vi "FTW-ActorTemplate.vi"(0 "FTW Actor Instance Configuration":string="{\n  \"Identity\": \"ActorName\",\n  \"InboxAddress\": \"inproc://*\",\n  \"LoggerAddress\": \"\",\n  \"DebugEnableInboxLogging\": false,\n  \"DebugEnableJobLogging\": false,\n  \"LauncherAddress\": \"\"\n}", 11 "ErrorIn":errorcluster) -> (15 "Error":errorcluster)   [LabVIEW 2015]
uses:
  source/actor/Instance/FTW-ActorInstance.lvclass
  source/actor/Message/Base/FTW-Message.lvclass
  source/actor/Instance/FTW-ActorInstance.lvclass/FTW-ActorInstance.ctl
  source/actor/JobSequencer/FTW-SEQ-Current.vi
  source/actor/Message/Request/FTW-Message-IncomingRequest.lvclass
panel:
  # "Inputs"
  # "Outputs"
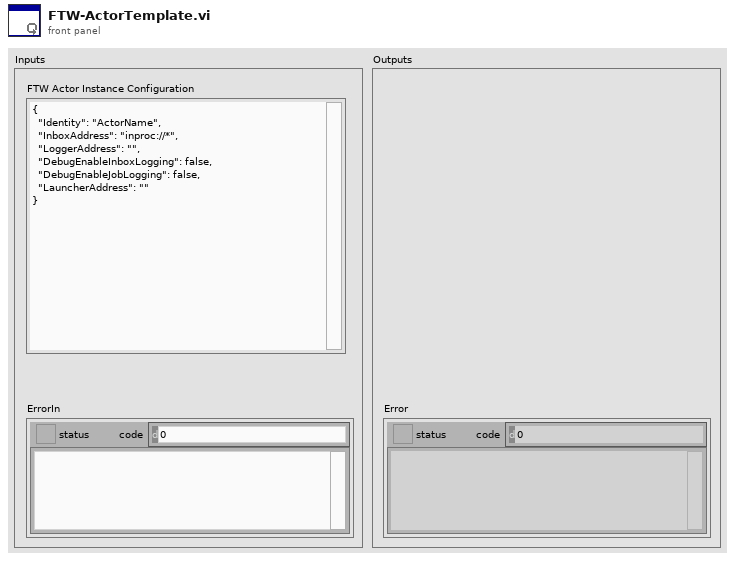
[diagram p1: front panel]
types:
  T1 = cluster{"Incoming Requests":refnum<event-registration>, "Local Messages":refnum<event-registration>, "Additional Registration Types":refnum<event-registration>}
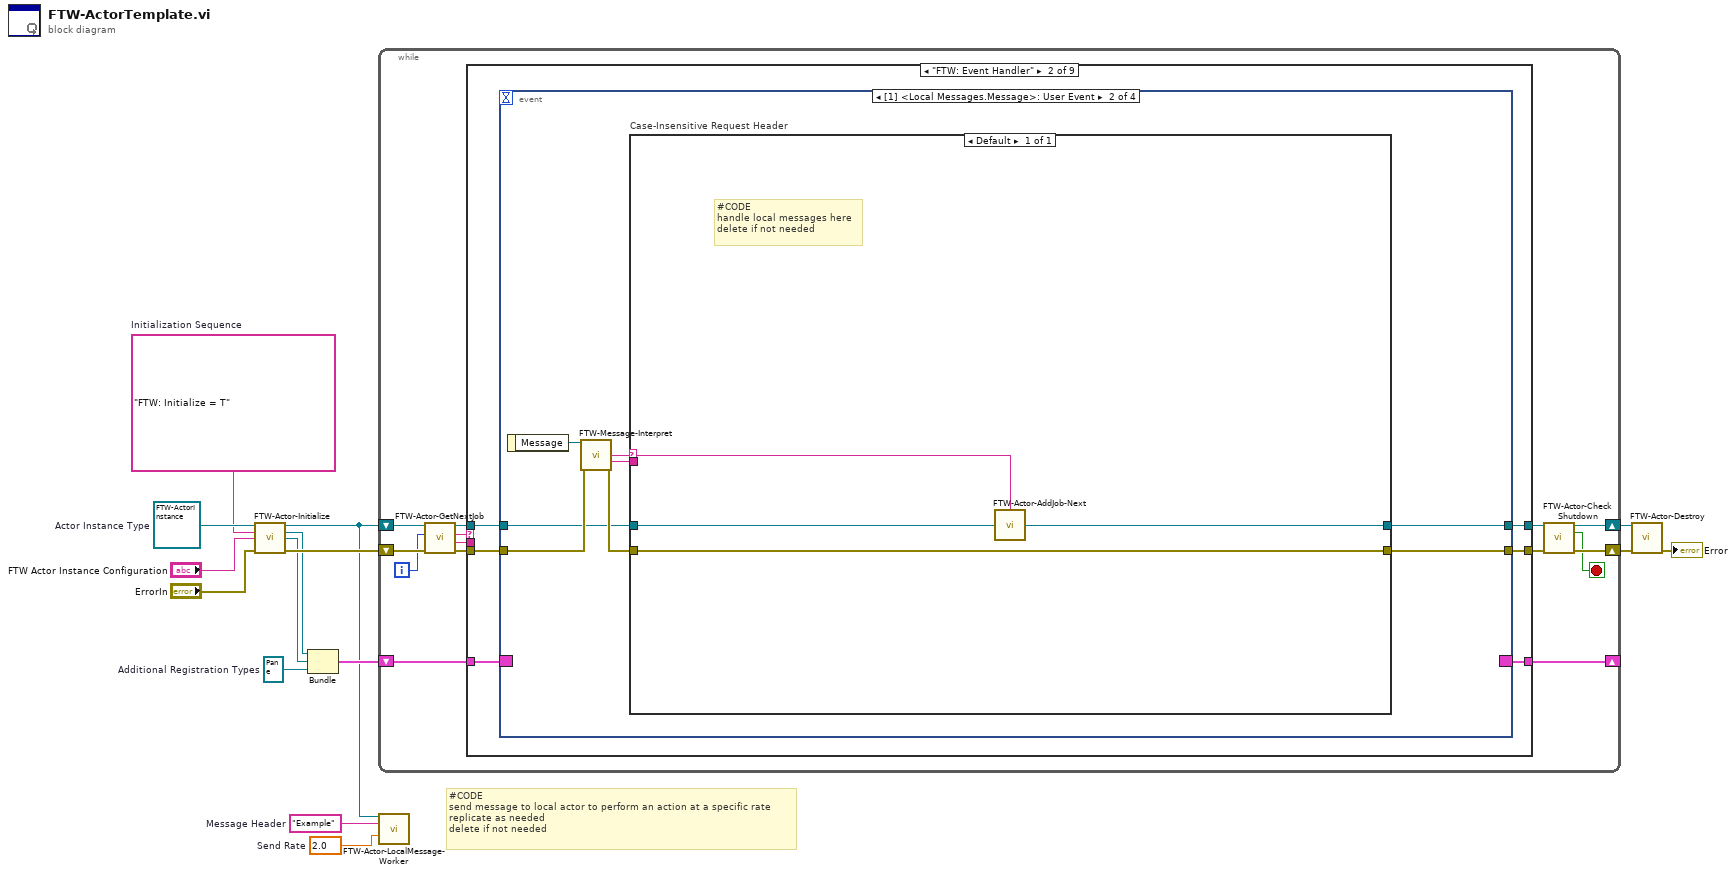
[diagram p0: block diagram]
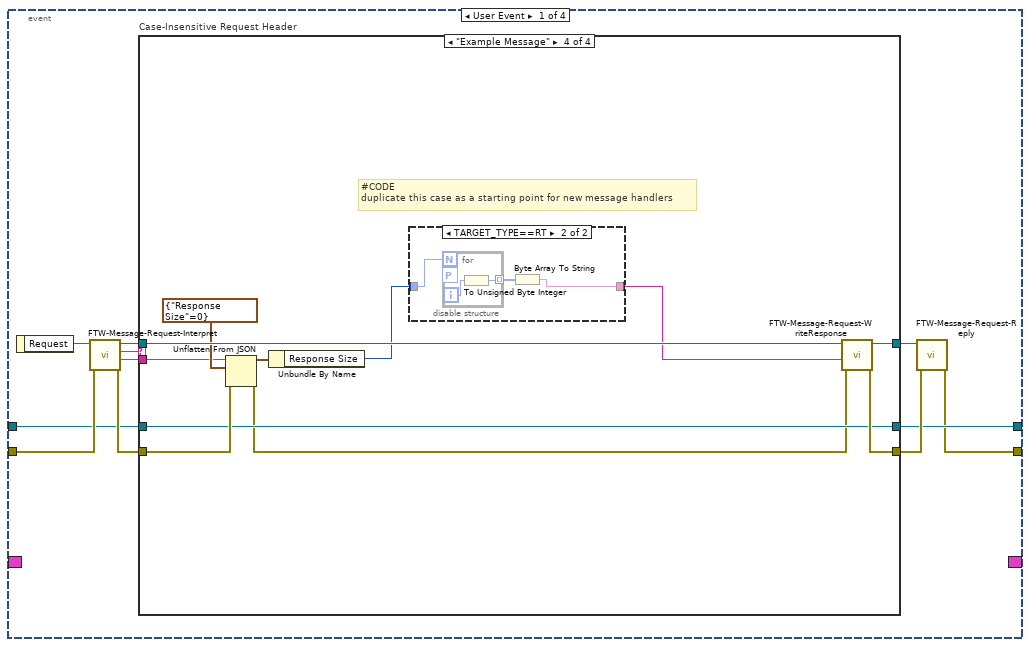
[diagram p3: hidden frame]
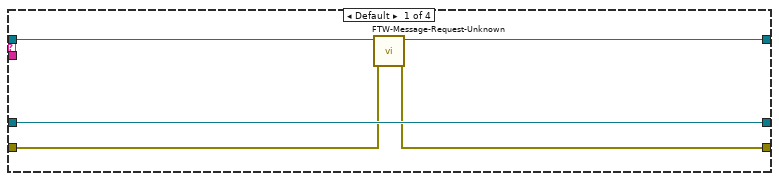
[diagram p4: hidden frame]
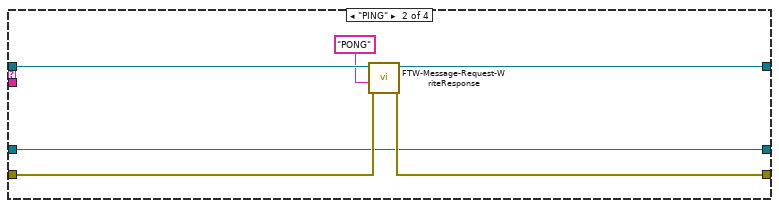
[diagram p5: hidden frame]
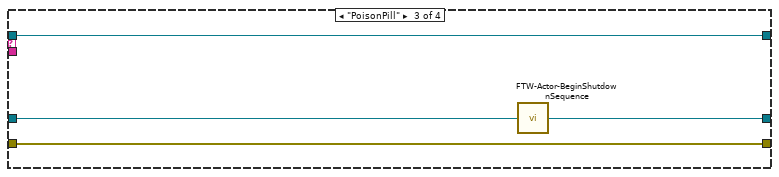
[diagram p6: hidden frame]
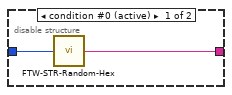
[diagram p7: hidden frame]
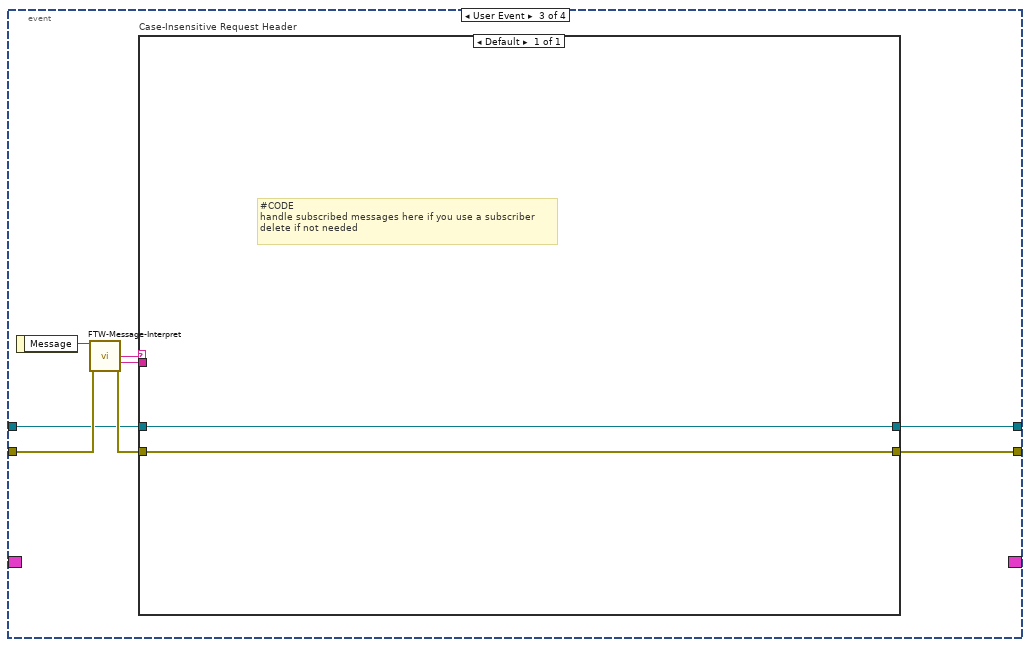
[diagram p8: hidden frame]
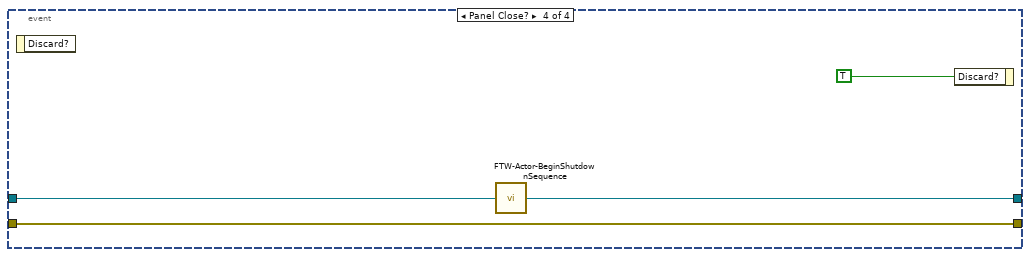
[diagram p9: hidden frame]
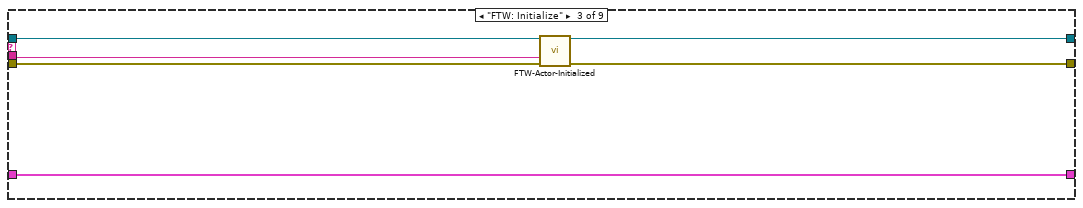
[diagram p10: hidden frame]
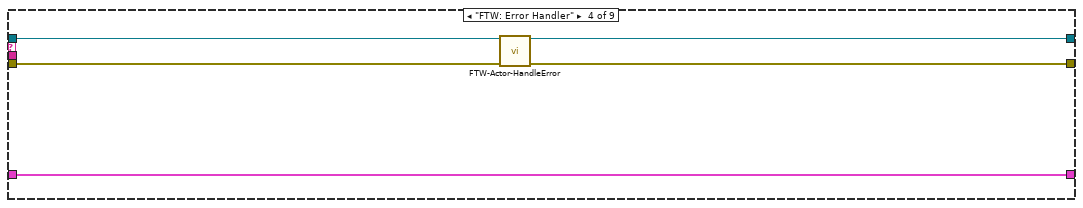
[diagram p11: hidden frame]
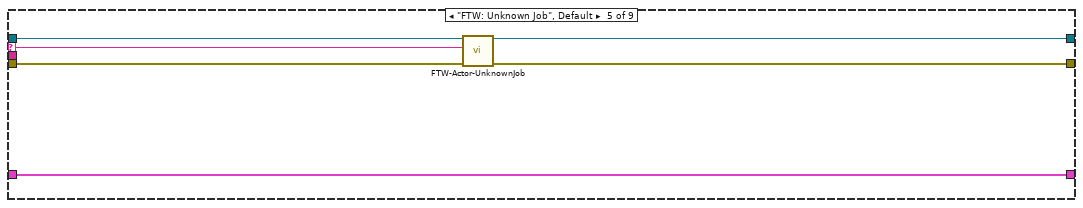
[diagram p12: hidden frame]
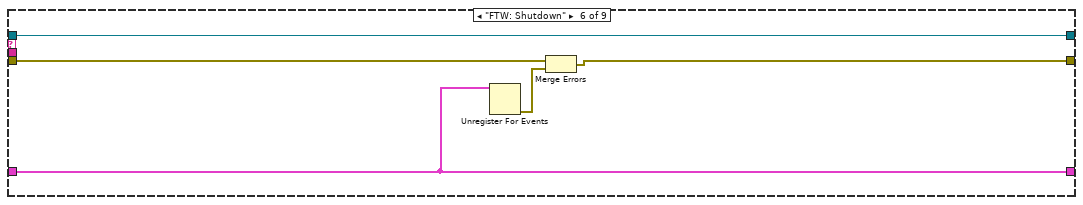
[diagram p13: hidden frame]
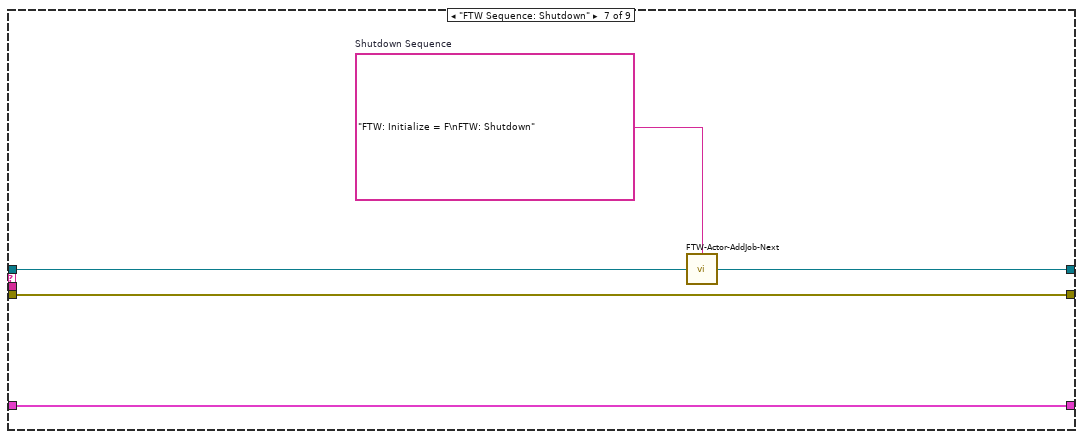
[diagram p14: hidden frame]
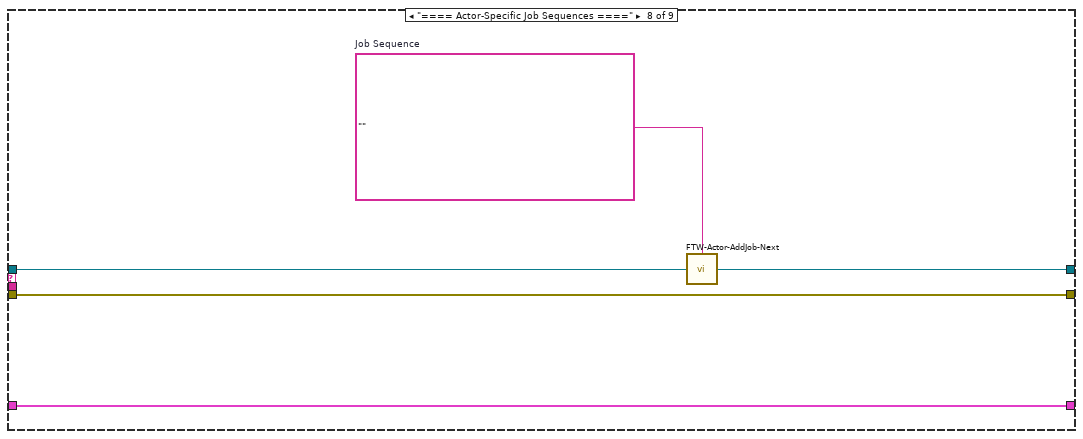
[diagram p15: hidden frame]
diagram:
  w1 = 2.0  # Send Rate
  w2 = "Example"  # Message Header
  w4 = refnum<event-registration> refnum  # Additional Registration Types
  w11 = refnum<class "FTW-ActorInstance.lvclass"> refnum  # Actor Instance Type
  w10 = "FTW: Initialize = T"  # Initialization Sequence
  # "#CODE\nsend message to local actor to perform an action at a specific rate\nreplicate as needed\ndelete if not needed"
  n1 = call-dynamic "FTW-Actor-Initialize.vi"("FTW Actor Instance Type"=w11, "Initialization Job Sequence"=w10, "Actor Instance Configuration"="FTW Actor Instance Configuration", "error in"="ErrorIn") -> ("FTW Actor Instance"=w3:refnum<class "FTW-ActorInstance.lvclass">, "Incoming Requests"=w6:refnum<event-registration>, "Local Messages"=w5:refnum<event-registration>, "error out"=w12:errorcluster)  [unwired: 8 in]
  n2 = Bundle("Incoming Requests"=w6, "Local Messages"=w5, "Additional Registration Types"=w4) -> (w8:T1)  [unwired: 1 in]
  n3 = while {
    shift-right: [w19] -> w14
    shift-left: w12 -> [w26]
    shift-right: [w16] -> _
    shift-left: w8 -> [w29]
    shift-right: [w21] -> w15
    shift-left: w3 -> [w28]
    i -> [w17]
    stop <- w18 stop-if-true
    n4 = call "FTW-Actor-GetNextJob.vi"("error in"=w26, "Jobs Performed"=w17, "FTW Actor Instance"=w28) -> ("error out"=w25:errorcluster, "Job Data"=w23:string, "Job Name"=w24:string, "FTW Actor Instance out"=w27:refnum<class "FTW-ActorInstance.lvclass">)  [unwired: 5 in]
    n5 = case shown="\"FTW: Event Handler\"" w24 {
      selector: w24 -> [_ _ _ _ w120 _ _ _ _]
      tunnel: [w31 w38 w110 w115 w123 w129 w134 w139 w143] -> w20
      tunnel: w25 -> [w31 w37 w113 w117 w124 w130 w134 w139 w143]
      tunnel: w29 -> [w32 w33 w114 w119 w125 w126 w135 w140 w142]
      tunnel: [w32 w36 w114 w119 w125 w126 w135 w140 w142] -> w16
      tunnel: w23 -> [_ _ w109 _ _ _ _ _ _]
      tunnel: [w30 w35 w111 w116 w121 w127 w132 w137 w141] -> w22
      tunnel: w27 -> [w30 w34 w112 w118 w122 w127 w133 w138 w141]
      frame "==== Featherweight Framework Jobs ====" {
      }
      frame "FTW: Event Handler" {
        n6 = event shown="[1] <Local Messages.Message>: User Event" {
          selector: w33 -> [_ _ _ _]
          dyn-events: [_ _ _ _] -> w36
          timeout: _ -> [_ _ _ _]
          tunnel: [w41 w87 w99 w107] -> w38
          tunnel: w37 -> [w47 w88 w100 w107]
          tunnel: [w45 w86 w98 w105] -> w35
          tunnel: w34 -> [w44 w85 w97 w106]
          event User Event {
            n7 = event-data() -> ("Request"=w48:refnum<class "FTW-Message-IncomingRequest.lvclass">)  [unwired: 1 in]
            n8 = call "FTW-Message-Request-Interpret.vi"("error in"=w47, "FTW Incoming Request"=w48) -> ("error out"=w49:errorcluster, "Request Body"=w39:string, "Request Header"=w43:string, "FTW Incoming Request out"=w42:refnum<class "FTW-Message-IncomingRequest.lvclass">)  [unwired: 6 in]
            n9 = case "Case-Insensitive Request Header" shown="\"Example Message\"" w43 {
              tunnel: [w52 w58 w63 w74] -> w46
              tunnel: w49 -> [w53 w59 w63 w75]
              tunnel: [w54 w57 w64 w71] -> w45
              tunnel: w44 -> [w54 w57 w62 w71]
              tunnel: w42 -> [w51 w60 w61 w73]
              tunnel: [w50 w56 w61 w72] -> w40
              tunnel: w39 -> [_ _ _ w65]
              frame Default {
                n10 = call "FTW-Message-Request-Unknown.vi"("error in"=w53, "FTW Incoming Request"=w51) -> ("error out"=w52:errorcluster, "FTW Incoming Request Out"=w50:refnum<class "FTW-Message-IncomingRequest.lvclass">)  [unwired: 8 in]
              }
              frame "PING" {
                n11 = call "FTW-Message-Request-WriteResponse.vi"("error in"=w59, "Response Body"="PONG" ("Response Header"), "FTW Incoming Request"=w60) -> ("error out"=w58:errorcluster, "FTW Incoming Request out"=w56:refnum<class "FTW-Message-IncomingRequest.lvclass">)  [unwired: 7 in]
              }
              frame "PoisonPill" {
                n12 = call "FTW-Actor-BeginShutdownSequence.vi"("FTW Actor Instance"=w62) -> ("FTW Actor Instance out"=w64:refnum<class "FTW-ActorInstance.lvclass">)  [unwired: 3 in]
              }
              frame "Example Message" {
                # "#CODE\nduplicate this case as a starting point for new message handlers"
                n13 = Unflatten From JSON(JSON string=w65, type and defaults=cluster{"Response Size":i32} {"Response Size"=0}, error in (no error)=w75) -> (value=w68:cluster{"Response Size":i32}, error out=w70:errorcluster)  [unwired: 4 in]
                n14 = Unbundle By Name(w68) -> ("Response Size"=w67:i32)
                n15 = disable-structure shown="TARGET_TYPE==RT" {
                  disable-tunnel: w67 -> [w77 w80]
                  disable-tunnel: [w76 w78] -> w66
                  frame condition #0 (active) {
                    n16 = call "FTW-STR-Random-Hex.vi"("String Length"=w77) -> ("Random Hex String"=w76:string)  [unwired: 3 in]
                  }
                  frame condition #1 {
                    n17 = for {
                      N: w80 -> [_]
                      workers-P: _ -> [_]
                      tunnel: [w81] -> w79 mode=indexing
                      i -> [w82]
                      n18 = To Unsigned Byte Integer(number=w82) -> (unsigned 8bit integer=w81:u8)
                    }
                    n19 = Byte Array To String(unsigned byte array=w79) -> (string=w78:string)
                  }
                }
                n20 = call "FTW-Message-Request-WriteResponse.vi"("error in"=w70, "Response Body"=w66, "FTW Incoming Request"=w73) -> ("error out"=w74:errorcluster, "FTW Incoming Request out"=w72:refnum<class "FTW-Message-IncomingRequest.lvclass">)  [unwired: 7 in]
              }
            }
            n21 = call "FTW-Message-Request-Reply.vi"("FTW: Reply Error"=w46, "FTW Incoming Request"=w40) -> ("error out"=w41:errorcluster)  [unwired: 8 in, 1 out]
          }
          event User Event {
            n22 = event-data() -> ("Message"=w89:refnum<class "FTW-Message.lvclass">)  [unwired: 1 in]
            n23 = call-dynamic "FTW-Message-Interpret.vi"("FTW Message"=w89, "error in"=w88) -> ("Message Header"=w83:string, "Message Body"=w84:string, "error out"=w90:errorcluster)  [unwired: 9 in, 2 out]
            n24 = case "Case-Insensitive Request Header" shown="Default" w83 {
              selector: w83 -> [w91]
              tunnel: [w93] -> w87
              tunnel: w90 -> [w93]
              tunnel: [w92] -> w86
              tunnel: w85 -> [w94]
              tunnel: w84 -> [_]
              frame Default {
                # "#CODE\nhandle local messages here\ndelete if not needed"
                n25 = call "FTW-Actor-AddJob-Next.vi"("Add Next in Job Queue"=w91, "FTW Actor Instance"=w94) -> ("FTW Actor Instance out"=w92:refnum<class "FTW-ActorInstance.lvclass">)  [unwired: 2 in]
              }
            }
          }
          event User Event {
            n26 = event-data() -> ("Message"=w101:refnum<class "FTW-Message.lvclass">)  [unwired: 1 in]
            n27 = call-dynamic "FTW-Message-Interpret.vi"("FTW Message"=w101, "error in"=w100) -> ("Message Header"=w95:string, "Message Body"=w96:string, "error out"=w102:errorcluster)  [unwired: 9 in, 2 out]
            n28 = case "Case-Insensitive Request Header" shown="Default" w95 {
              tunnel: [w103] -> w99
              tunnel: w102 -> [w103]
              tunnel: [w104] -> w98
              tunnel: w97 -> [w104]
              tunnel: w96 -> [_]
              frame Default {
                # "#CODE\nhandle subscribed messages here if you use a subscriber\ndelete if not needed"
              }
            }
          }
          event Panel Close? {
            n29 = event-data() -> ()  [unwired: 1 in, 1 out]
            n30 = call "FTW-Actor-BeginShutdownSequence.vi"("FTW Actor Instance"=w106) -> ("FTW Actor Instance out"=w105:refnum<class "FTW-ActorInstance.lvclass">)  [unwired: 3 in]
            n31 = event-data("Discard?"=TRUE) -> ()  [unwired: 1 in, 1 out]
          }
        }
      }
      frame "FTW: Initialize" {
        n32 = call-dynamic "FTW-Actor-Initialized.vi"("FTW Actor Instance"=w112, "Positive Init?"=w109, "error in"=w113) -> ("FTW Actor Instance out"=w111:refnum<class "FTW-ActorInstance.lvclass">, "error out"=w110:errorcluster)  [unwired: 11 in]
      }
      frame "FTW: Error Handler" {
        n33 = call-dynamic "FTW-Actor-HandleError.vi"("FTW Actor Instance"=w118, "error in"=w117) -> ("FTW Actor Instance out"=w116:refnum<class "FTW-ActorInstance.lvclass">, "error out"=w115:errorcluster)  [unwired: 10 in, 2 out]
      }
      frame "FTW: Unknown Job", Default {
        n34 = call-dynamic "FTW-Actor-UnknownJob.vi"("FTW Actor Instance"=w122, "Unknown Job"=w120, "error in"=w124) -> ("FTW Actor Instance out"=w121:refnum<class "FTW-ActorInstance.lvclass">, "error out"=w123:errorcluster)  [unwired: 11 in]
      }
      frame "FTW: Shutdown" {
        n35 = Unregister For Events(event registration refnum=w126) -> (error out=w128:errorcluster)  [unwired: 1 in]
        n36 = Merge Errors(w130, w128) -> (w129:errorcluster)
      }
      frame "FTW Sequence: Shutdown" {
        w131 = "FTW: Initialize = F\nFTW: Shutdown"  # Shutdown Sequence
        n37 = call "FTW-Actor-AddJob-Next.vi"("Add Next in Job Queue"=w131, "FTW Actor Instance"=w133) -> ("FTW Actor Instance out"=w132:refnum<class "FTW-ActorInstance.lvclass">)  [unwired: 2 in]
      }
      frame "==== Actor-Specific Job Sequences ====" {
        w136 = ""  # Job Sequence
        n38 = call "FTW-Actor-AddJob-Next.vi"("Add Next in Job Queue"=w136, "FTW Actor Instance"=w138) -> ("FTW Actor Instance out"=w137:refnum<class "FTW-ActorInstance.lvclass">)  [unwired: 2 in]
      }
      frame "==== Actor-Specific Jobs ====" {
      }
    }
    n39 = call "FTW-Actor-CheckShutdown.vi"("FTW Actor Instance"=w22, "error in"=w20) -> ("FTW Actor Instance out"=w21:refnum<class "FTW-ActorInstance.lvclass">, "Shutdown?"=w18:bool, "error out"=w19:errorcluster)  [unwired: 11 in]
  }
  n40 = call-dynamic "FTW-Actor-LocalMessage-Worker.vi"("FTW-ActorInstance In"=w3, "Message Header"=w2, "Send Rate"=w1) -> ()  [unwired: 13 in]
  n41 = call-dynamic "FTW-Actor-Destroy.vi"("FTW Actor Instance"=w15, "error in"=w14) -> ("error out"=→"Error":errorcluster)  [unwired: 13 in]
